vi "GlobalWhereAmI.vi"() -> ()   [LabVIEW 2012]
doc: "This Global variable contains where the robot curretnly is as well as its direction"
panel:
  out "WhereAmI?":T1
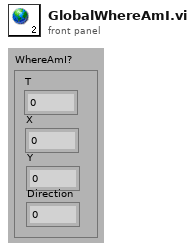
[diagram p1: front panel]
types:
  T1 = cluster{"T":dbl, "X":dbl, "Y":dbl, "Direction":dbl}
diagram:
